vi "helioscan settings to tag settings.vi"(10 "scan specification - helioscan":T2) -> (2 "scan specification - tag resonant":T1)   [LabVIEW 2010]
uses:
  scan_specification_cluster.ctl
  scan_specification_tagResonant.ctl
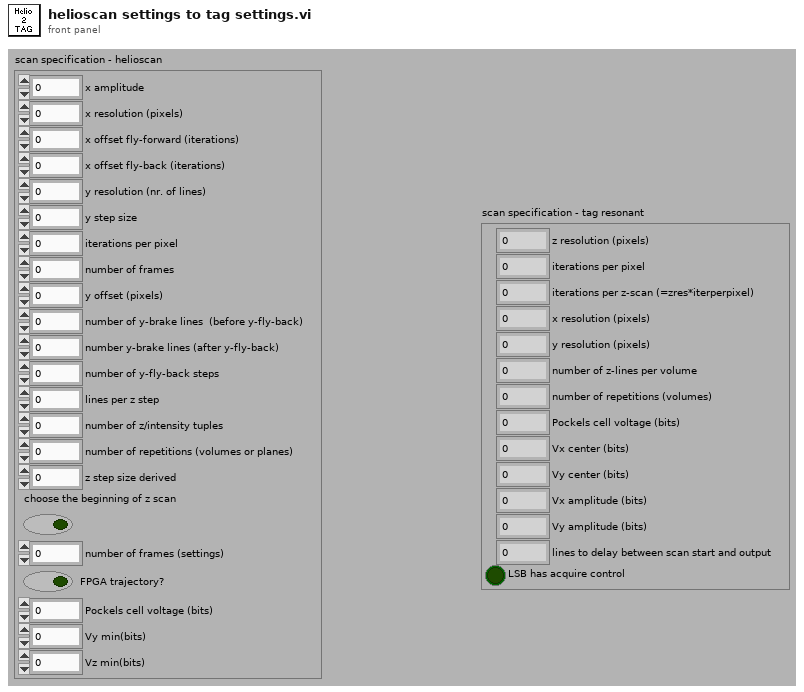
[diagram p1: front panel]
types:
  T1 = typedef "scan_specification_tagResonant.ctl" = cluster{"z resolution (pixels)":u16, "iterations per pixel":u16, "iterations per z-scan (=zres*iterperpixel)":u16, "x resolution (pixels)":u16, "y resolution (pixels)":u16, "number of z-lines per volume":u16, "number of repetitions (volumes)":i32, "Pockels cell voltage (bits)":i16, "Vx center (bits)":i16, "Vy center (bits)":i16, "Vx amplitude (bits)":i16, "Vy amplitude (bits)":i16, "lines to delay between scan start and output":u16, "LSB has acquire control":bool}
  T2 = typedef "scan_specification_cluster.ctl" = cluster{"x amplitude":u16, "x resolution (pixels)":u16, "x offset fly-forward (iterations)":u16, "x offset fly-back (iterations)":u16, "y resolution (nr. of lines)":u16, "y step size":u16, "iterations per pixel":u16, "number of frames":i32, "y offset (pixels)":u16, "number of y-brake lines  (before y-fly-back)":u16, "number y-brake lines (after y-fly-back)":u16, "number of y-fly-back steps":u16, "lines per z step":u16, "number of z/intensity tuples":u16, "number of repetitions (volumes or planes)":i32, "z step size derived":u16, "choose the beginning of z scan":bool, "number of frames (settings)":i32, "FPGA trajectory?":bool, "Pockels cell voltage (bits)":i16, "Vy min(bits)":i16, "Vz min(bits)":i16}
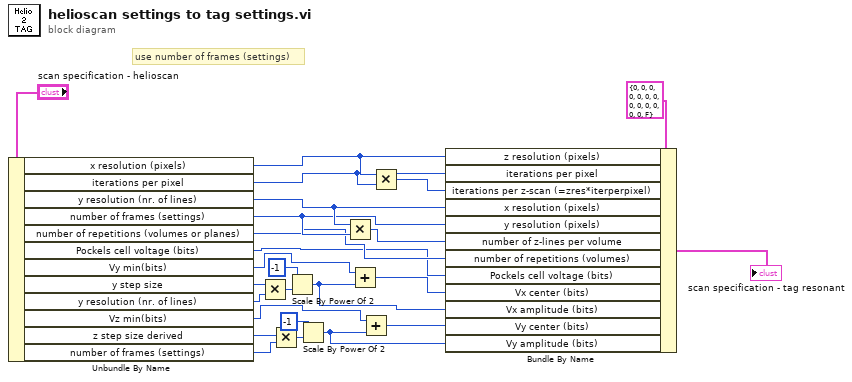
[diagram p0: block diagram]
diagram:
  # "use number of frames (settings)"
  n1 = Unbundle By Name("scan specification - helioscan") -> ("x resolution (pixels)"=w22:u16, "iterations per pixel"=w21:u16, "y resolution (nr. of lines)"=w19:u16, "number of frames (settings)"=w18:i32, "number of repetitions (volumes or planes)"=w16:i32, "Pockels cell voltage (bits)"=w15:i16, "Vy min(bits)"=w9:i16, "y step size"=w14:u16, "y resolution (nr. of lines)"=w13:u16, "Vz min(bits)"=w3:i16, "z step size derived"=w5:u16, "number of frames (settings)"=w4:i32)
  n2 = Multiply(x=w14, y=w13) -> (x*y=w12:u16)
  n3 = Multiply(x=w5, y=w4) -> (x*y=w7:i32)
  n4 = Scale By Power Of 2(n=-1, x=w12) -> (x*2^n=w10:u16)
  n5 = Scale By Power Of 2(n=-1, x=w7) -> (x*2^n=w1:i32)
  n6 = Multiply(x=w19, y=w18) -> (x*y=w17:i32)
  n7 = Add(x=w9, y=w10) -> (x+y=w8:u16)
  n8 = Add(x=w3, y=w1) -> (x+y=w2:i32)
  n9 = Multiply(x=w22, y=w21) -> (x*y=w20:u16)
  n10 = Bundle By Name(cluster=T1 {"z resolution (pixels)"=0, "iterations per pixel"=0, "iterations per z-scan (=zres*iterperpixel)"=0, "x resolution (pixels)"=0, "y resolution (pixels)"=0, "number of z-lines per volume"=0, "number of repetitions (volumes)"=0, "Pockels cell voltage (bits)"=0, "Vx center (bits)"=0, "Vy center (bits)"=0, "Vx amplitude (bits)"=0, "Vy amplitude (bits)"=0, "lines to delay between scan start and output"=0, "LSB has acquire control"=FALSE} ("scan specification - tag resonant"), "z resolution (pixels)"=w22, "iterations per pixel"=w21, "iterations per z-scan (=zres*iterperpixel)"=w20, "x resolution (pixels)"=w19, "y resolution (pixels)"=w18, "number of z-lines per volume"=w17, "number of repetitions (volumes)"=w16, "Pockels cell voltage (bits)"=w15, "Vx center (bits)"=w8, "Vx amplitude (bits)"=w10, "Vy center (bits)"=w2, "Vy amplitude (bits)"=w1) -> (→"scan specification - tag resonant":T1)
